vi "sweep_finished.vi"(8 "error in (no error)":errorcluster, 11 "DataCollectionDL091104Scaffold in":refnum<class "DataCollectionDL091104Scaffold.lvclass">) -> (0 "error out":errorcluster, 3 "DataCollectionDL091104Scaffold out":refnum<class "DataCollectionDL091104Scaffold.lvclass">)   [LabVIEW 2010, in "DataCollectionDL091104Scaffold.lvclass"]
uses:
  DataCollectionDL091104Scaffold.lvclass
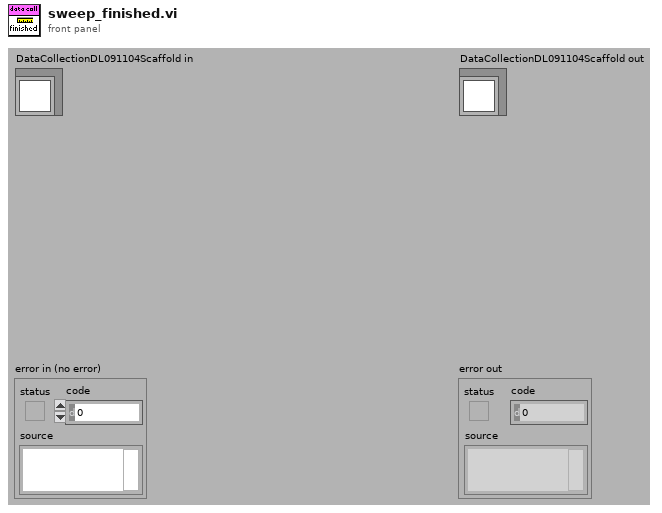
[diagram p1: front panel]
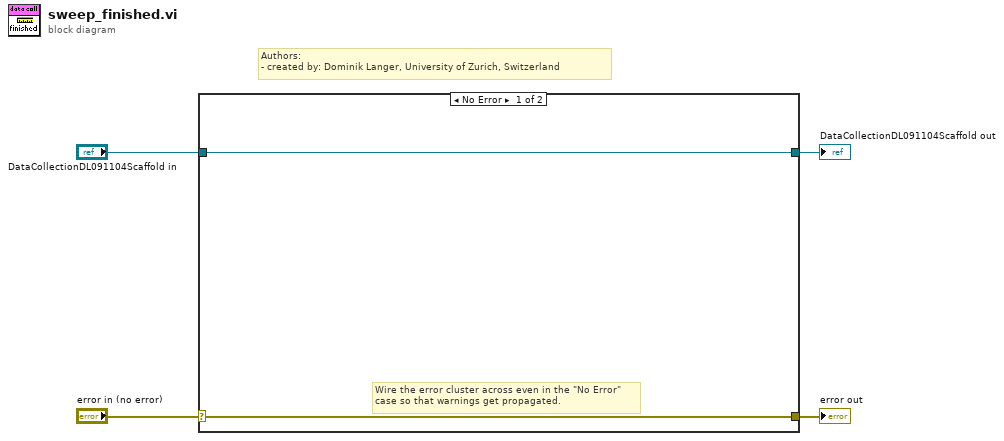
[diagram p0: block diagram]
diagram:
  # "Authors: \n- created by: Dominik Langer, University of Zurich, Switzerland"
  n1 = case shown="No Error" "error in (no error)" {
    selector: "error in (no error)" -> [w5 w8]
    tunnel: [w5 w8] -> w3
    tunnel: [w6 w7] -> w1
    tunnel: "DataCollectionDL091104Scaffold in" -> [w6 w7]
    frame No Error {
      # "Wire the error cluster across even in the \"No Error\"\ncase so that warnings get propagated."
    }
    frame Error {
    }
  }
  "error out" <- w3
  "DataCollectionDL091104Scaffold out" <- w1
